vi "Periodic Tasks.vi"(8 "error in":errorcluster) -> ()   [LabVIEW 2016]
doc: "This VI runs in parallel to other tasks. It can contain as many user-defined periodic loops as you need. These can carry out PID or other sorts of timed response."
uses:
  <vilib>/Rock Robotics/WPI/Utilities/WPI_GetSetVariantRefNum.vi
  <vilib>/Rock Robotics/Network Tables/NT Write Number.vi
  <vilib>/Instr/_visa.llb/VISA Configure Serial Port (Instr).vi
  Systems/Global 1.vi
  Global 2.vi
panel:
  out "LD Encoder Velocity":dbl
  out "RD Encoder Velocity":dbl
  in  "Gyro Reset":bool
  out "Angle":dbl=-21.734980684494005
  in  "Reset Drive":bool
  out "Waveform Chart":dbl(graph)=-10000.0
  out "PSI":dbl=-12.426759099999998
  out "Shoot 0":dbl format="%#_13g"
  out "Shoot 1":dbl format="%#_13g"
  out "read buffer":string="B:0,X:-3,Y:-3,W1:-3,H1:-3,W2:-3,H2:-3\r\n"
  in  "Search_Params":string[](array[string])=["B", "X", "Y", "W1", "H1", "W2", "H2"]
  out "Last Complete Message":string="B:0,X:-3,Y:-3,W1:-3,H1:-3,W2:-3,H2:-3"
  out "length":i32=37
  in  "off set":dbl format="%#_13g"
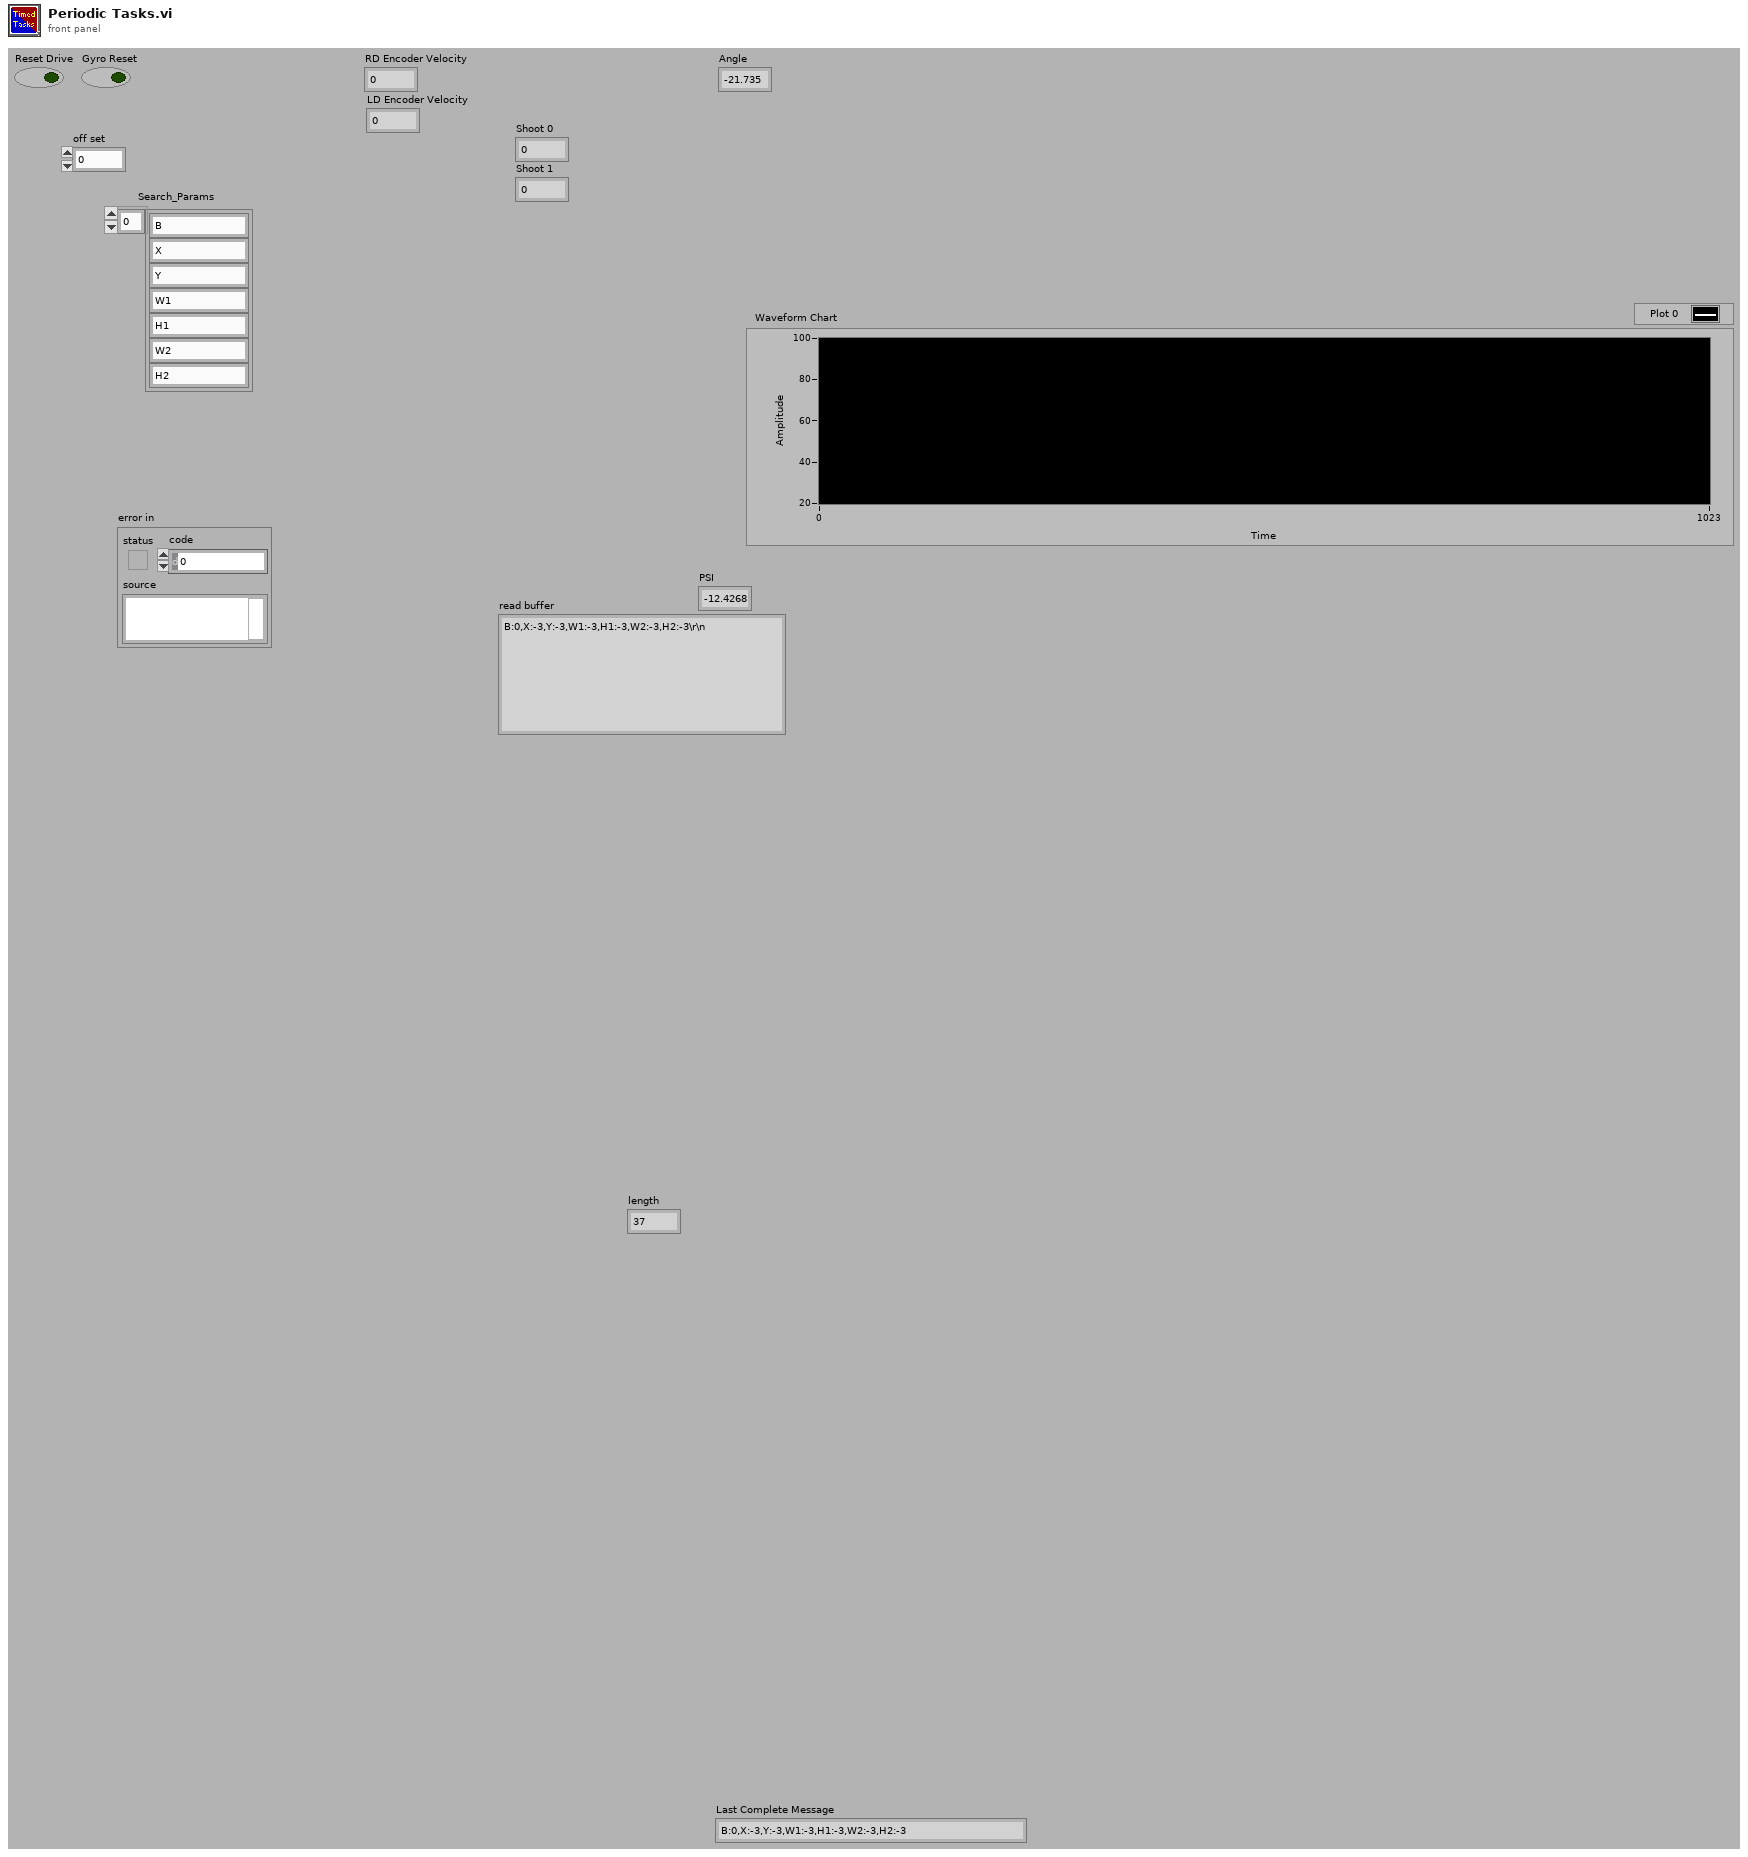
[diagram p1: front panel]
types:
  T1 = typedef "WPI_JoystickDevRef.ctl" = cluster{"Device":T2}
  T2 = typedef "WPI_JoystickDeviceEnum.ctl" = enum16{"USB 0", "USB 1", "USB 2", "USB 3", "USB 4", "USB 5"}
  T3 = typedef "WPI_MotorControlDeviceRef.ctl" = cluster{"DeviceStatus":errorcluster, "Type":T4, "PWM":cluster{"PWM Channel":T5, "DeadBand":T6}, "CAN":cluster{"Device Number":u8, "SetOutput VI Ref":variant, "GetOutput VI Ref":variant, "Enable VI Ref":variant, "Disable VI Ref":variant, "Data":variant}, "Invert":bool}
  T4 = typedef "WPI_MotorControlType.ctl" = enum16{"PWM", "CAN"}
  T5 = typedef "FPGA_DIOPWMChannel.ctl" = enum8{"PWM 0", "PWM 1", "PWM 2", "PWM 3", "PWM 4", "PWM 5", "PWM 6", "PWM 7", "PWM 8", "PWM 9", "PWM MXP 0", "PWM MXP 1", "PWM MXP 2", "PWM MXP 3", "PWM MXP 4", "PWM MXP 5", "PWM MXP 6", "PWM MXP 7", "PWM MXP 8", "PWM MXP 9", "Invalid"}
  T6 = typedef "WPI_PWMDeadband.ctl" = cluster{"Name":string, "maxPositivePwm":i32, "minPositivePwm":i32, "centerPwm":i32, "maxNegativePwm":i32, "minNegativePwm":i32, "angularRange":u16}
  T7 = typedef "WPI_CANTalonSRX_GlobalStatus.ctl" = cluster{"Applied Throttle":dbl, "Module Enabled":bool, "CAN Error":errorcluster, "Closed Loop Error":dbl, "Forward Limit Switch Closed":bool, "Reverse Limit Switch Closed":bool, "Sensor Position":dbl, "Sensor Velocity":dbl, "Current":dbl, "Sticky Fault - Over Temp":bool, "Sticky Fault - Under Voltage":bool, "Sticky Fault - Forward Limit":bool, "Sticky Fault - Reverse Limit":bool, "Sticky Fault - Forward Soft Limit":bool, "Sticky Fault - Reverse Soft Limit":bool, "Brake is Enabled":bool, "Encoder Position":dbl, "Encoder Velocity":dbl, "Encoder Index Count":dbl, "Encoder A Pin State":bool, "Encoder B Pin State":bool, "Encoder Index Pin State":bool, "Analog In":dbl, "Analog In Velocity":dbl, "Temperature (C)":dbl, "Battery Voltage":dbl, "Control 5 Is Supported":bool, "Current Profile Slot Select":dbl, "Pos Div 8":bool, "Vel Div 4":bool, "Pulse Width Position":i32, "Pulse Width Velocity":i32, "Pulse Width Rise To Rise (us)":i32, "Pulse Width Rise To Fall (us)":i32, "Mot Prof Active Is Under Run":bool, "Mot Prof Active Has Under Run":bool, "Mot Prof Active Is Last":bool, "Mot Prof Active Velocity Only":bool, "Mot Prof Active Is Valid":bool, "Mot Prof Buffer Is Full":bool, "Mot Prof Active Profile Slot Select":i32, "Mot Prof NextID":i32, "Mot Prof Count":i32, "Mot Prof Active Velocity":dbl, "Mot Prof Active Position":dbl, "Mot Prof Output Enable":i32}
  T8 = typedef "WPI_AnalogChannelDevRef.ctl" = cluster{"DevStatus":errorcluster, "Analog Channel":T9}
  T9 = typedef "FPGA_AIChannel.ctl" = enum8{"AI 0", "AI 1", "AI 2", "AI 3", "AI MXP 0", "AI MXP 1", "AI MXP 2", "AI MXP 3", "Invalid"}
  T10 = typedef "WPI_GyroDevRef.ctl" = cluster{"DevStatus":errorcluster, "Analog Channel":T9, "Offset":dbl, "Gain (VoltsPerDegree/Second)":dbl, "Gyro Type":enum16{"Analog", "XRS450"}, "Handle":i32, "SPI Bus":T11, "Device Found":bool, "Sample Rate":dbl, "Calibrate On Open":bool}
  T11 = typedef "spi_bus.ctl" = enum16{"SPI On-Board, CS0", "SPI On-Board, CS1", "SPI On-Board, CS2", "SPI On-Board, CS3", "SPI MXP", "Invalid"}
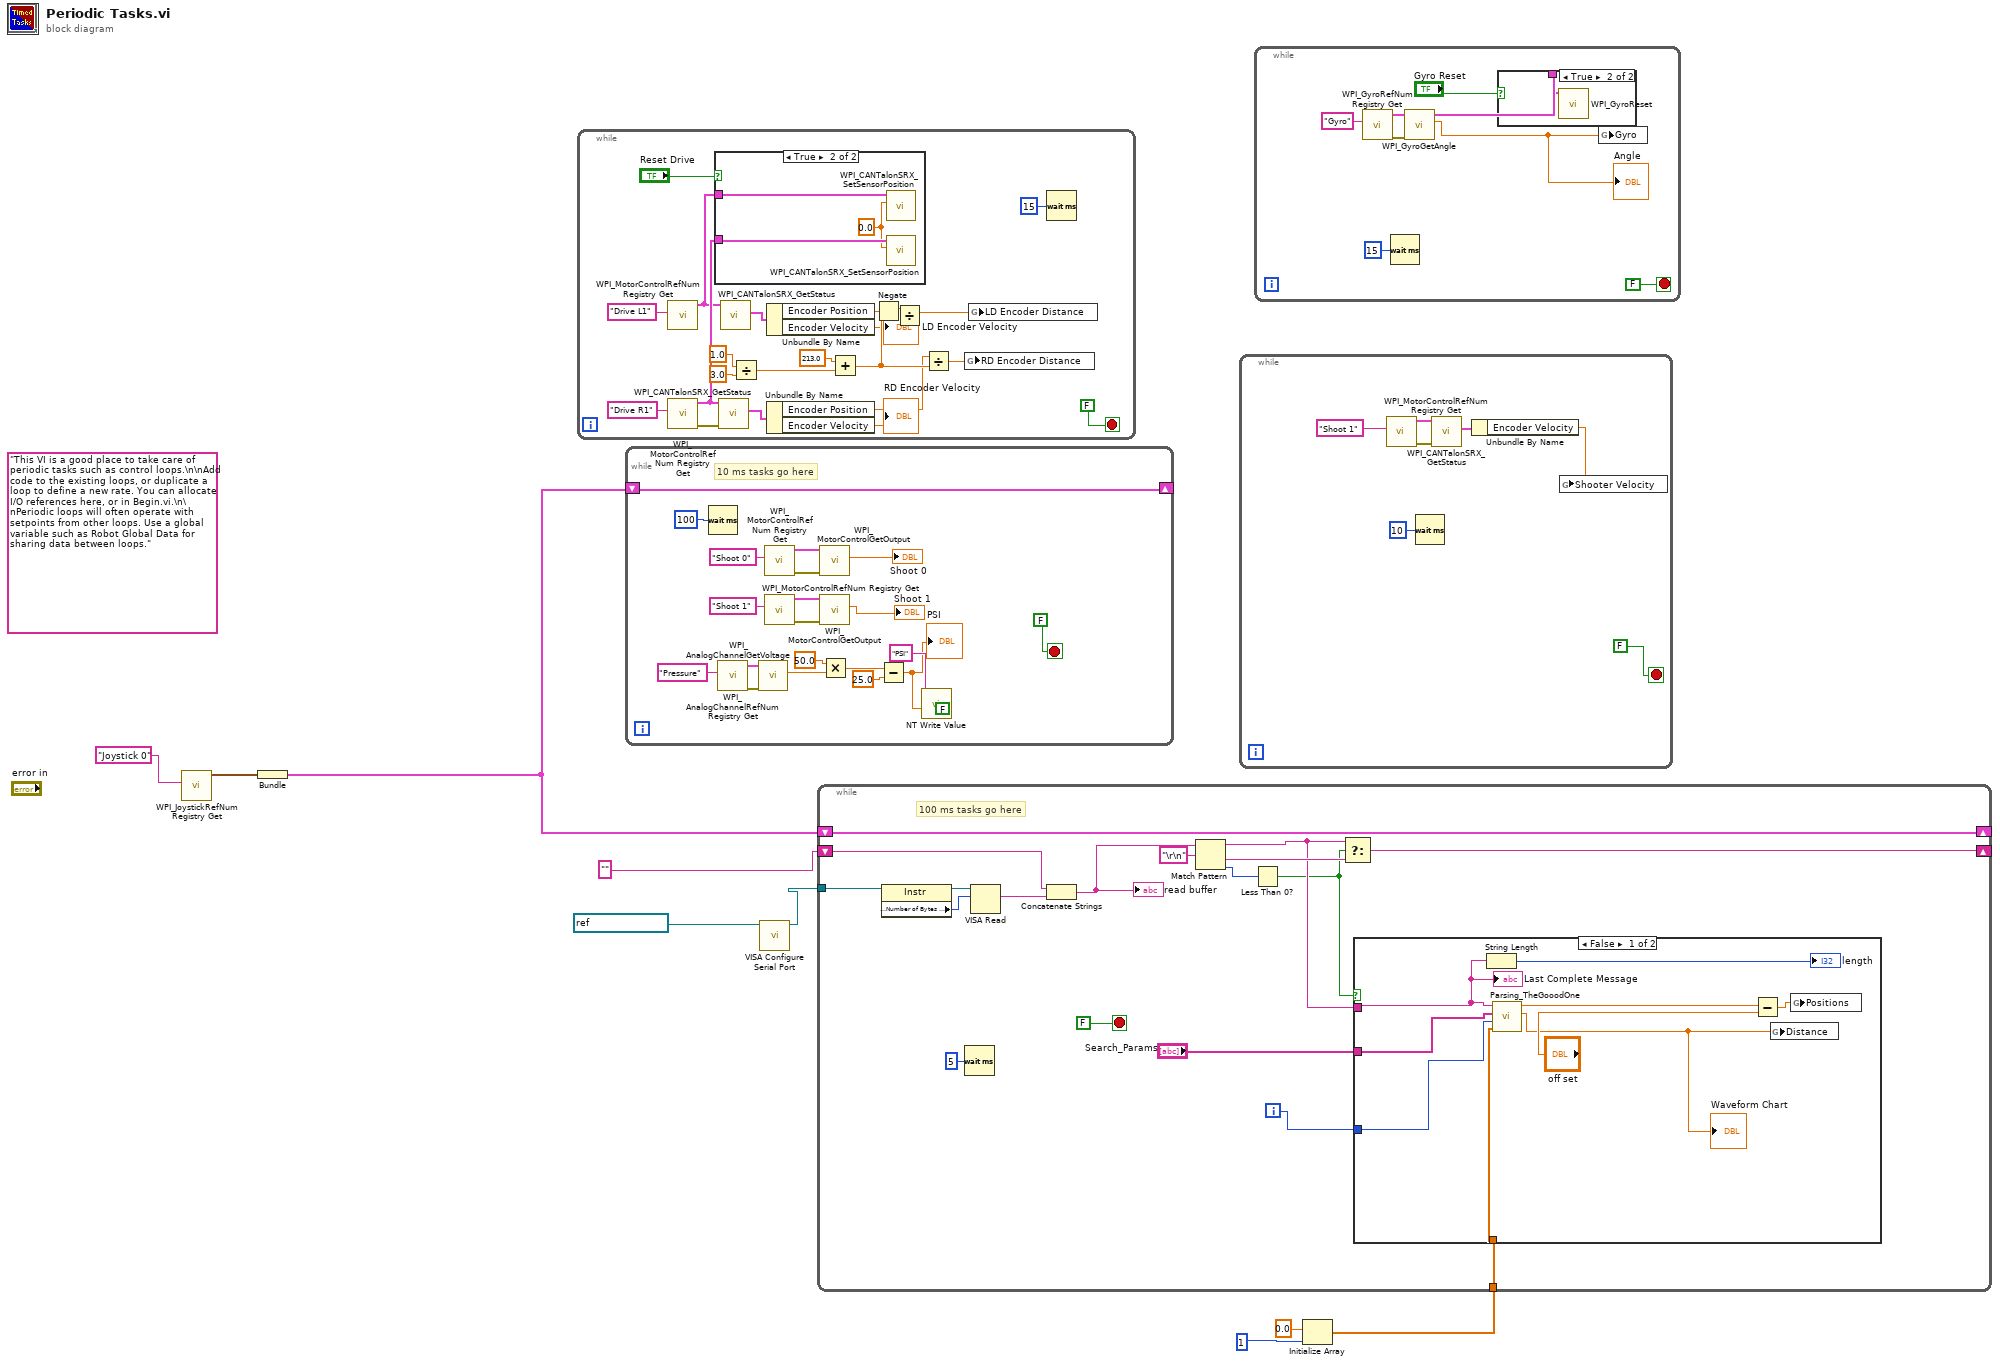
[diagram p0: block diagram]
diagram:
  (unwired) "This VI is a good place to take care of periodic tasks such as control loops.\n\nAdd code to the existing loops, or duplicate a loop to define a new rate. You can allocate I/O references here, or in Begin.vi.\n\nPeriodic loops will often operate with setpoints from other loops. Use a global variable such as Robot Global Data for sharing data between loops."
  n1 = call <vilib>:"WPI_JoystickRefNum Registry Get.vi"("refnum name"="Joystick 0") -> ("JoystickDevRef"=w2:T1)  [unwired: 1 in, 9 out]
  n2 = Bundle("JoystickDevRef"=w2) -> (w3:cluster{"JoystickDevRef":T1})  [unwired: 1 out]
  n3 = while {
    stop <- FALSE stop-if-true
    n4 = call <vilib>:"WPI_MotorControlRefNum Registry Get.vi"("refnum name"="Drive L1") -> ("MotorControlDevRef"=w24:T3)  [unwired: 9 in, 1 out]
    n5 = call <vilib>:"WPI_MotorControlRefNum Registry Get.vi"("refnum name"="Drive R1") -> ("error out"=w29:errorcluster, "MotorControlDevRef"=w25:T3)  [unwired: 9 in]
    n6 = case shown="True" "Reset Drive" {
      tunnel: w25 -> [_ w34]
      tunnel: w24 -> [_ w33]
      frame False {
      }
      frame True {
        w32 = 0.0
        n7 = call <vilib>:"WPI_CANTalonSRX_SetSensorPosition.vi"("New Sensor Position"=w32, "CAN Talon SRX Ref"=w33) -> ()  [unwired: 8 in, 2 out]
        n8 = call <vilib>:"WPI_CANTalonSRX_SetSensorPosition.vi"("New Sensor Position"=w32, "CAN Talon SRX Ref"=w34) -> ()  [unwired: 8 in, 2 out]
      }
    }
    n9 = call <vilib>:"WPI_CANTalonSRX_GetStatus.vi"("error in (no error)"=w29, "CAN Talon SRX Ref"=w25) -> ("Talon SRX Status"=w30:T7)  [unwired: 7 in, 2 out]
    n10 = call <vilib>:"WPI_CANTalonSRX_GetStatus.vi"("CAN Talon SRX Ref"=w24) -> ("Talon SRX Status"=w27:T7)  [unwired: 8 in, 2 out]
    n11 = Divide(x=1.0, y=3.0) -> (x/y=w20:dbl)
    n12 = Unbundle By Name(w27) -> ("Encoder Position"=w18:dbl, "Encoder Velocity"=→"LD Encoder Velocity":dbl)
    n13 = Unbundle By Name(w30) -> ("Encoder Position"=w14:dbl, "Encoder Velocity"=→"RD Encoder Velocity":dbl)
    n14 = Add(x=213.0, y=w20) -> (x+y=w17:dbl)
    n15 = Negate(x=w18) -> (-x=w12:dbl)
    n16 = Divide(x=w12, y=w17) -> (x/y=w13:dbl)
    n17 = Divide(x=w14, y=w17) -> (x/y=w16:dbl)
    n18 = global write "Global 2.vi" "RD Encoder Distance"(w16) -> ()
    n19 = global write "Global 2.vi" "LD Encoder Distance"(w13) -> ()
    n20 = Wait (ms)(milliseconds to wait=u32 15) -> ()  [unwired: 1 out]
  }
  n21 = while {
    shift-right: [w52] -> _
    shift-left: w3 -> [w52]
    stop <- FALSE stop-if-true
    (unwired) FALSE
    # "10 ms tasks go here"
    n22 = Wait (ms)(milliseconds to wait=u32 100) -> ()  [unwired: 1 out]
    n23 = call <vilib>:"WPI_AnalogChannelRefNum Registry Get.vi"("refnum name"="Pressure") -> ("error out"=w43:errorcluster, "AIDeviceRef"=w42:T8)  [unwired: 9 in]
    n24 = call <vilib>:"WPI_AnalogChannelGetVoltage.vi"("error in (no error)"=w43, "AIDeviceRef"=w42) -> ("Voltage"=w40:dbl)  [unwired: 7 in, 2 out]
    n25 = call <vilib>:"WPI_MotorControlRefNum Registry Get.vi"("refnum name"="Shoot 0") -> ("error out"=w47:errorcluster, "MotorControlDevRef"=w51:T3)  [unwired: 9 in]
    n26 = call <vilib>:"WPI_MotorControlRefNum Registry Get.vi"("refnum name"="Shoot 1") -> ("error out"=w46:errorcluster, "MotorControlDevRef"=w48:T3)  [unwired: 9 in]
    n27 = call <vilib>:"WPI_MotorControlGetOutput.vi"("error in"=w47, "MotorControlDevRef"=w51) -> ("Output"=→"Shoot 0":dbl)  [unwired: 7 in, 2 out]
    n28 = call <vilib>:"WPI_MotorControlGetOutput.vi"("error in"=w46, "MotorControlDevRef"=w48) -> ("Output"=→"Shoot 1":dbl)  [unwired: 7 in, 2 out]
    n29 = Multiply(x=50.0, y=w40) -> (x*y=w38:dbl)
    n30 = Subtract(x=w38, y=25.0) -> (x-y=w35:dbl)
    "PSI" <- w35
    n31 = call-poly <vilib>:"NT Write Value.vi"("Numeric"=w35, "Name"="PSI") -> ()  [unwired: 9 in, 1 out]
  }
  n32 = call-poly "VISA Configure Serial Port"("VISA resource name"=refnum<visa-resource-name> "ASRL2::INSTR") -> ("VISA resource name out"=w5:refnum<visa-resource-name>)  [unwired: 13 in, 1 out]
  n33 = while {
    stop <- FALSE stop-if-true
    n34 = call <vilib>:"WPI_MotorControlRefNum Registry Get.vi"("refnum name"="Shoot 1") -> ("error out"=w59:errorcluster, "MotorControlDevRef"=w60:T3)  [unwired: 9 in]
    n35 = Wait (ms)(milliseconds to wait=u32 10) -> ()  [unwired: 1 out]
    n36 = call <vilib>:"WPI_CANTalonSRX_GetStatus.vi"("error in (no error)"=w59, "CAN Talon SRX Ref"=w60) -> ("Talon SRX Status"=w58:T7)  [unwired: 7 in, 2 out]
    n37 = Unbundle By Name(w58) -> ("Encoder Velocity"=w57:dbl)
    n38 = global write "Global 2.vi" "Shooter Velocity"(w57) -> ()
  }
  n39 = while {
    stop <- FALSE stop-if-true
    n40 = call <vilib>:"WPI_GyroRefNum Registry Get.vi"("refnum name"="Gyro") -> ("error out"=w66:errorcluster, "GyroDevRef"=w69:T10)  [unwired: 9 in]
    n41 = Wait (ms)(milliseconds to wait=u32 15) -> ()  [unwired: 1 out]
    n42 = call <vilib>:"WPI_GyroGetAngle.vi"("error in"=w66, "GyroDevRef"=w69) -> ("Angle"=w63:dbl, "GyroDevRef"=w65:T10)  [unwired: 5 in, 3 out]
    "Angle" <- w63
    n43 = case shown="True" "Gyro Reset" {
      tunnel: w65 -> [_ w70]
      frame False {
      }
      frame True {
        n44 = call <vilib>:"WPI_GyroReset.vi"("GyroDevRef"=w70) -> ()  [unwired: 9 in, 2 out]
      }
    }
    n45 = global write "Global 2.vi" "Gyro"(w63) -> ()
  }
  n46 = Initialize Array(0.0 ("element"), 1) -> (w9:dbl[])
  n47 = while {
    shift-right: [w87] -> _
    shift-left: w3 -> [w87]
    tunnel: w5 -> [w82]
    shift-right: [w74] -> _
    shift-left: "" -> [w81]
    tunnel: w9 -> [w71]
    i -> [w72]
    stop <- FALSE stop-if-true
    # "100 ms tasks go here"
    n48 = property class="Instr"(reference=w82) -> (reference out=w86:refnum<visa-resource-name>, "Serial Settings:Number of Bytes at Serial Port"=w85:u32)  [unwired: 1 in, 1 out]
    n49 = Wait (ms)(milliseconds to wait=u32 5) -> ()  [unwired: 1 out]
    n50 = VISA Read(VISA resource name=w86, byte count=w85) -> (read buffer=w80:string)  [unwired: 1 in, 3 out]
    n51 = Concatenate Strings(w81, w80) -> (w79:string)
    "read buffer" <- w79
    n52 = Match Pattern(string=w79, regular expression="\r\n") -> (before substring=w75:string, after substring=w76:string, offset past match=w77:i32)  [unwired: 1 in, 1 out]
    n53 = Less Than 0?(x=w77) -> (x < 0?=w73:bool)
    n54 = Select(t=w75, s=w73, f=w76) -> (s? t:f=w74:string)
    n55 = case shown="False" w73 {
      tunnel: "Search_Params" -> [w96 _]
      tunnel: w75 -> [w95 _]
      tunnel: w72 -> [w91 _]
      tunnel: w71 -> [w90 _]
      frame False {
        n56 = String Length(string=w95) -> (length=→"length":i32)
        n57 = call "Parsing_TheGooodOne.vi"("array"=w90, "Iterations"=w91, "Search_Params"=w96, "Input"=w95) -> ("Corrected distance"=w89:dbl, "Value-Reference"=w94:dbl)  [unwired: 4 in]
        "Waveform Chart" <- w89
        n58 = Subtract(x=w94, y="off set") -> (x-y=w92:dbl)
        n59 = global write "Global 1.vi" "Distance"(w89) -> ()
        n60 = global write "Global 1.vi" "Positions"(w92) -> ()
        "Last Complete Message" <- w95
      }
      frame True {
      }
    }
  }
